vi "GV-LegendMouseOver.vi"(6 "Origin":cluster{"x":i16, "y":i16}, 8 "error in (no error)":errorcluster, 9 "Coords":T1, 11 "Gviewer in":refnum<class "Gviewer.lvclass">) -> (0 "error out":errorcluster, 1 "image":picture, 3 "Gviewer out":refnum<class "Gviewer.lvclass">)   [LabVIEW 2020, in "Sgraph_lib_V1.lvlib" / "Gviewer.lvclass"]
doc: "Andre Koelewijn, 27 April 2021\n\nActions when mouse hovers over Legend Area"
uses:
  Gviewer.lvclass
  <vilib>/Utility/miscctls.llb/LVPoint32TypeDef.ctl
  Gviewer.lvclass/Gviewer.ctl
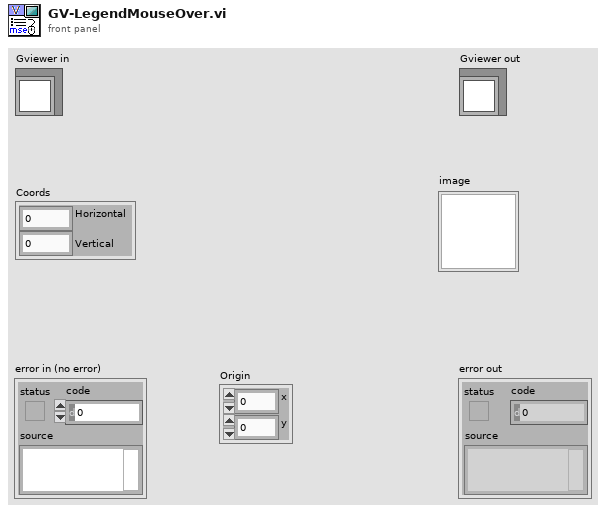
[diagram p1: front panel]
types:
  T1 = typedef "LVPoint32TypeDef.ctl" = cluster{"Horizontal":i32, "Vertical":i32}
  T2 = cluster{"horizontal":enum16{"left", "center", "right"}, "vertical":enum16{"top", "center", "bottom"}}
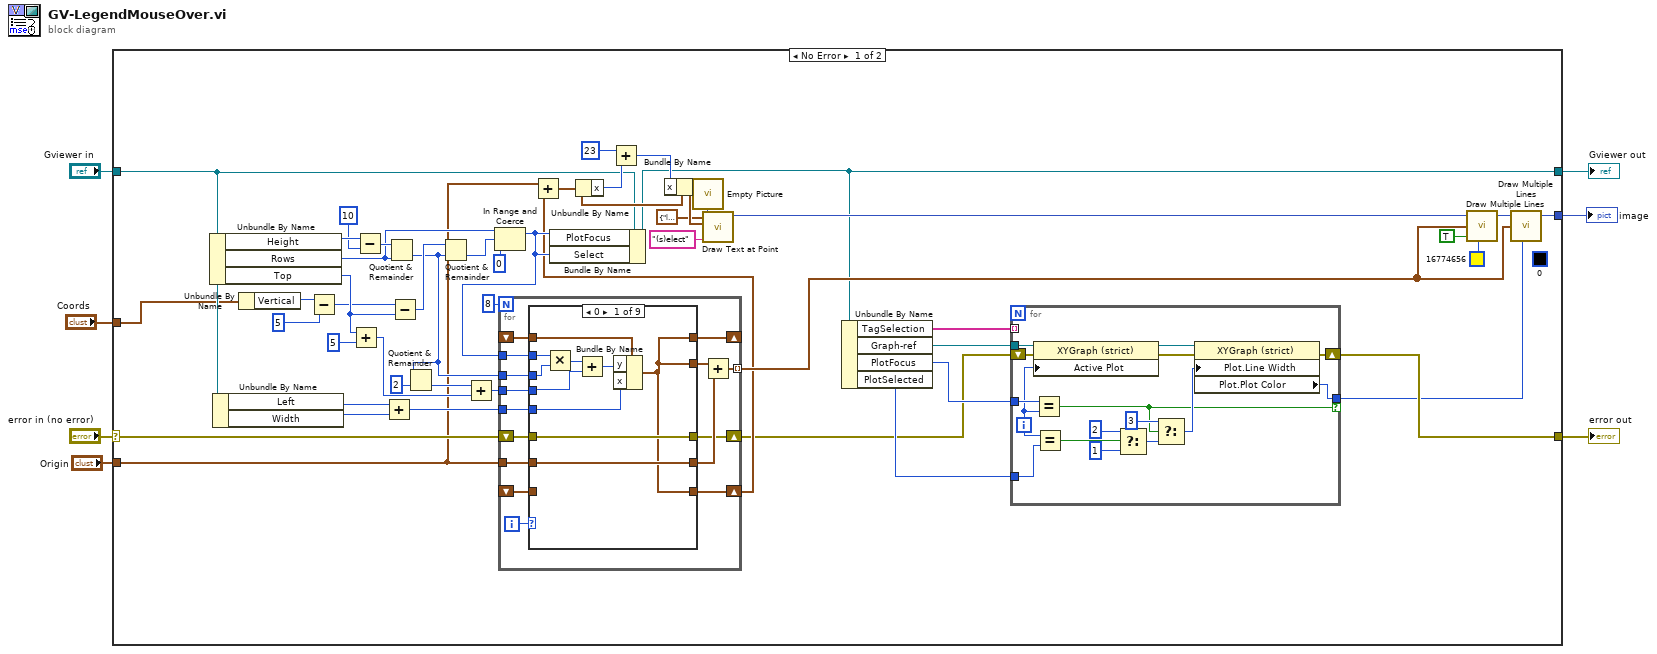
[diagram p0: block diagram]
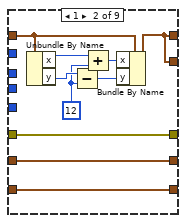
[diagram p2: hidden frame]
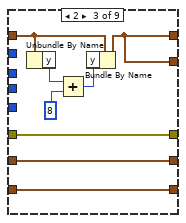
[diagram p3: hidden frame]
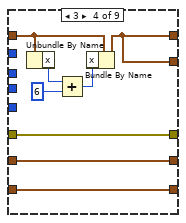
[diagram p4: hidden frame]
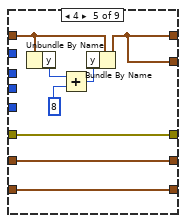
[diagram p5: hidden frame]
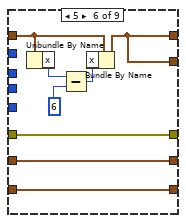
[diagram p6: hidden frame]
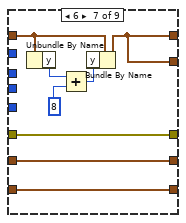
[diagram p7: hidden frame]
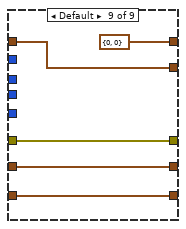
[diagram p9: hidden frame]
diagram:
  n1 = case shown="No Error" "error in (no error)" {
    selector: "error in (no error)" -> [w19 w157]
    tunnel: [w10 w157] -> w6
    tunnel: [w15 w156] -> w4
    tunnel: "Gviewer in" -> [w21 w156]
    tunnel: "Coords" -> [w20 _]
    tunnel: "Origin" -> [w18 _]
    tunnel: [w17 _] -> w2
    frame No Error {
      (unwired) u32 0
      # "``"
      n2 = Unbundle By Name(w21) -> ("Height"=w44:u32, "Rows"=w36:u32, "Top"=w41:i32)
      n3 = Unbundle By Name(w21) -> ("Left"=w51:i32, "Width"=w50:u32)
      n4 = Unbundle By Name(w20) -> ("Vertical"=w34:i32)
      n5 = Subtract(x=w34, y=5) -> (x-y=w32:i32)
      n6 = Add(x=w41, y=5) -> (x+y=w39:i32)
      n7 = Subtract(x=w44, y=u32 10) -> (x-y=w42:u32)
      n8 = Add(x=w51, y=w50) -> (x+y=w49:u32)
      n9 = Quotient & Remainder(x=w42, y=w36) -> (floor(x/y)=w48:u32)  [unwired: 1 out]
      n10 = Subtract(x=w32, y=w41) -> (x-y=w56:i32)
      n11 = Quotient & Remainder(x=w48, y=u32 2) -> (floor(x/y)=w46:u32)  [unwired: 1 out]
      n12 = Quotient & Remainder(x=w56, y=w48) -> (floor(x/y)=w38:u32)  [unwired: 1 out]
      n13 = Add(x=w46, y=w39) -> (x+y=w45:u32)
      n14 = In Range and Coerce(upper limit=w36, x=w38, lower limit=u32 0) -> (coerced(x)=w35:u32)  [unwired: 1 out]
      n15 = for {
        N: 8 -> [_]
        shift-right: [w82] -> w11
        shift-left: w19 -> [w83]
        tunnel: w18 -> [w85]
        tunnel: [w87] -> w53 mode=indexing
        tunnel: w35 -> [w81]
        tunnel: w48 -> [w76]
        shift-right: [w80] -> _
        shift-left: _ -> [w79]
        tunnel: w49 -> [w77]
        tunnel: w45 -> [w75]
        shift-right: [w74] -> w24
        shift-left: _ -> [w73]
        i -> [w86]
        n16 = case shown="0" w86 {
          tunnel: w85 -> [w97 w102 w109 w117 w125 w133 w141 w149 w155]
          tunnel: [w97 w102 w109 w117 w125 w133 w141 w149 w155] -> w84
          tunnel: w83 -> [w96 w103 w110 w118 w126 w134 w142 w150 w154]
          tunnel: [w96 w103 w110 w118 w126 w134 w142 w150 w154] -> w82
          tunnel: w81 -> [w93 _ _ _ _ _ _ _ _]
          tunnel: [w88 w104 w111 w119 w127 w135 w143 w148 cluster{"x":i16, "y":i16} {"x"=0, "y"=0}] -> w80
          tunnel: w79 -> [w95 w107 w115 w123 w131 w139 w147 _ w152]
          tunnel: [w88 w104 w111 w119 w127 w135 w143 w148 w152] -> w78
          tunnel: w77 -> [w94 _ _ _ _ _ _ _ _]
          tunnel: w76 -> [w92 _ _ _ _ _ _ _ _]
          tunnel: w75 -> [w89 _ _ _ _ _ _ _ _]
          tunnel: [w88 w98 w108 w116 w124 w132 w140 w148 w151] -> w74
          tunnel: w73 -> [_ w98 w108 w116 w124 w132 w140 w148 w151]
          frame 0 {
            n17 = Multiply(x=w93, y=w92) -> (x*y=w91:u32)
            n18 = Add(x=w91, y=w89) -> (x+y=w90:u32)
            n19 = Bundle By Name(cluster=w95, "y"=w90, "x"=w94) -> (w88:cluster{"x":i16, "y":i16})
          }
          frame 1 {
            w99 = i16 12 ("y")
            n20 = Unbundle By Name(w107) -> ("x"=w106:i16, "y"=w101:i16)
            n21 = Subtract(x=w101, y=w99) -> (x-y=w100:i16)
            n22 = Add(x=w106, y=w99) -> (x+y=w105:i16)
            n23 = Bundle By Name(cluster=w107, "x"=w105, "y"=w100) -> (w104:cluster{"x":i16, "y":i16})
          }
          frame 2 {
            n24 = Unbundle By Name(w115) -> ("y"=w114:i16)
            n25 = Add(x=w114, y=i16 8) -> (x+y=w113:i16)
            n26 = Bundle By Name(cluster=w115, "y"=w113) -> (w111:cluster{"x":i16, "y":i16})
          }
          frame 3 {
            n27 = Unbundle By Name(w123) -> ("x"=w122:i16)
            n28 = Add(x=w122, y=i16 6) -> (x+y=w121:i16)
            n29 = Bundle By Name(cluster=w123, "x"=w121) -> (w119:cluster{"x":i16, "y":i16})
          }
          frame 4 {
            n30 = Unbundle By Name(w131) -> ("y"=w130:i16)
            n31 = Add(x=w130, y=i16 8) -> (x+y=w129:i16)
            n32 = Bundle By Name(cluster=w131, "y"=w129) -> (w127:cluster{"x":i16, "y":i16})
          }
          frame 5 {
            n33 = Unbundle By Name(w139) -> ("x"=w138:i16)
            n34 = Subtract(x=w138, y=i16 6) -> (x-y=w137:i16)
            n35 = Bundle By Name(cluster=w139, "x"=w137) -> (w135:cluster{"x":i16, "y":i16})
          }
          frame 6 {
            n36 = Unbundle By Name(w147) -> ("y"=w146:i16)
            n37 = Add(x=w146, y=i16 8) -> (x+y=w145:i16)
            n38 = Bundle By Name(cluster=w147, "y"=w145) -> (w143:cluster{"x":i16, "y":i16})
          }
          frame 7 {
          }
          frame Default {
          }
        }
        n39 = Add(x=w78, y=w84) -> (x+y=w87:cluster{"x":i16, "y":i16})
      }
      n40 = Add(x=w18, y=w24) -> (x+y=w23:cluster{"x":i16, "y":i16})
      n41 = Bundle By Name(cluster=w21, "PlotFocus"=w35, "Select"=w35) -> (w15:refnum<class "Gviewer.lvclass">)
      n42 = Unbundle By Name(w23) -> ("x"=w28:i16)
      n43 = Add(x=i16 23, y=w28) -> (x+y=w26:i16)
      n44 = Bundle By Name(cluster=w23, "x"=w26) -> (w27:cluster{"x":i16, "y":i16})
      n45 = call "Empty Picture"() -> ("empty picture"=w31:picture)
      n46 = call <vilib>:"Draw Text at Point.vi"("text"="(s)elect", "alignment(left, top)"=T2 {"horizontal"=enum."left", "vertical"=enum."center"}, "origin"=w27, "picture"=w31) -> ("new picture"=w30:picture)  [unwired: 6 in, 1 out]
      n47 = Unbundle By Name(w15) -> ("TagSelection"=w16:string[], "Graph-ref"=w12:refnum<vi>, "PlotFocus"=w13:i32, "PlotSelected"=w14:i32)
      n48 = for {
        tunnel: w16 -> [_] mode=indexing
        tunnel: w13 -> [w64]
        tunnel: [w57] -> w9 if=w65
        tunnel: w12 -> [w72]
        shift-right: [w66] -> w10
        shift-left: w11 -> [w68]
        tunnel: w14 -> [w61]
        i -> [w62]
        n49 = property class="XYGraph (strict)"(reference=w72, error in=w68, "Active Plot"=w62) -> (reference out=w71:refnum<vi>, error out=w67:errorcluster)
        n50 = Equal?(x=w64, y=w62) -> (x = y?=w65:bool)
        n51 = Equal?(x=w62, y=w61) -> (x = y?=w60:bool)
        n52 = Select(t=u8 2 ("Plot.Line Width"), s=w60, f=u8 1 ("Plot.Line Width")) -> (s? t:f=w63:u8)
        n53 = Select(t=u8 3 ("Plot.Line Width"), s=w65, f=w63) -> (s? t:f=w69:u8)
        n54 = property class="XYGraph (strict)"(reference=w71, error in=w67, "Plot.Line Width"=w69) -> (error out=w66:errorcluster, "Plot.Plot Color"=w57:u32)  [unwired: 1 out]
      }
      n55 = call <vilib>:"Draw Multiple Lines.vi"("picture"=w30, "line endpoints"=w53, "fill?(F)"=TRUE, "color(black)"=u32 16774656) -> ("new picture"=w54:picture)  [unwired: 5 in]
      n56 = call <vilib>:"Draw Multiple Lines.vi"("picture"=w54, "line endpoints"=w53, "color(black)"=w9) -> ("new picture"=w17:picture)  [unwired: 6 in]
    }
    frame Error {
    }
  }
  "error out" <- w6
  "Gviewer out" <- w4
  "image" <- w2
